vi "Write Common Config.vi"(8 "error in (no error)":errorcluster, 10 "Common":T1={"Period (s)"=0.001, "Offset (us)"=0, "ClockID"=0, "Priority"=100, "Processor"=-2} {"Period (s)" format="%#_13g"}, 11 "CIFTemplateNode in":refnum<class "CIFCorePlugin.lvclass">) -> (0 "error out":errorcluster, 3 "CIFTemplateNode out":refnum<class "CIFCorePlugin.lvclass">)   [LabVIEW 2021, in "CIFCorePlugin.lvclass"]
uses:
  CIFCorePlugin.lvclass
  Common/Typedef/Common Plugin Configuration.ctl
  CIFCorePlugin.lvclass/CIFCorePlugin.ctl
  CIFUtilities/CIFClocks/Time Conversion/LabVIEW Time to UTC Time.vi
  Common/Utilities/Add Error.vi
  Common/Utilities/Append Error Location.vi
  CIFUtilities/CIFClocks/CIFClocks.lvlib
  Common/CIFCoreCommon.lvlib
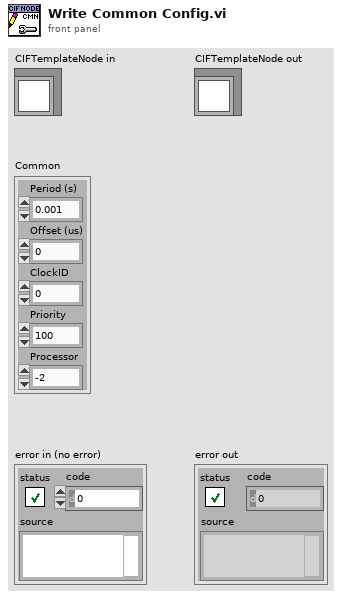
[diagram p1: front panel]
types:
  T1 = typedef "CIFCoreCommon.lvlib/Common Plugin Configuration.ctl" = cluster{"Period (s)":dbl, "Offset (us)":i32, "ClockID":u8, "Priority":i32, "Processor":i32}
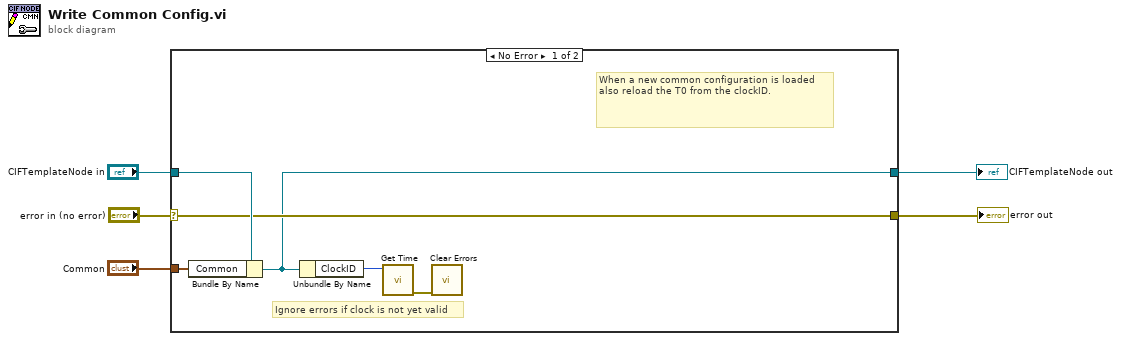
[diagram p0: block diagram]
diagram:
  n1 = case shown="No Error" "error in (no error)" {
    selector: "error in (no error)" -> [w7 w12]
    tunnel: [w7 w12] -> w4
    tunnel: [w6 w13] -> w2
    tunnel: "CIFTemplateNode in" -> [w11 w13]
    tunnel: "Common" -> [w10 _]
    frame No Error {
      # "Ignore errors if clock is not yet valid"
      # "When a new common configuration is loaded also reload the T0 from the clockID."
      n2 = Bundle By Name(cluster=w11, "Common"=w10) -> (w6:refnum<class "CIFCorePlugin.lvclass">)
      n3 = Unbundle By Name(w6) -> ("ClockID"=w8:u8)
      n4 = call "Get Time.vi"("ClockID"=w8) -> ("error out"=w9:errorcluster)  [unwired: 8 in, 2 out]
      n5 = call <vilib>:"Clear Errors.vi"("error in (no error)"=w9) -> ()  [unwired: 5 in, 2 out]
    }
    frame Error {
    }
  }
  "error out" <- w4
  "CIFTemplateNode out" <- w2
